vi "QTrkCheckForDLL.vi"   [LabVIEW 2011]
uses:
  QTrkDLL.vi
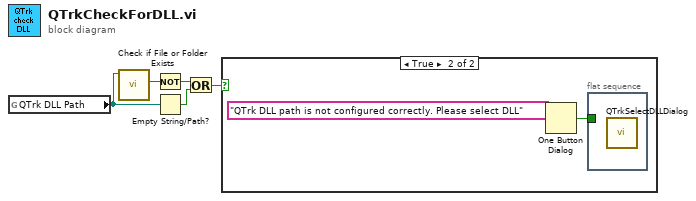
[diagram p0: block diagram]
diagram:
  n1 = global read "QTrkDLL.vi" "QTrk DLL Path"() -> (w5:path)
  n2 = call <vilib>:"Check if File or Folder Exists.vi"("path"=w5) -> ("file or folder exists?"=w3:bool)  [unwired: 8 in, 2 out]
  n3 = Not(x=w3) -> (.not. x?=w2:bool)
  n4 = Empty String/Path?(string/path=w5) -> (empty?=w1:bool)
  n5 = Or(x=w2, y=w1) -> (x .or. y?=w4:bool)
  n6 = case shown="True" w4 {
    frame False {
    }
    frame True {
      n7 = One Button Dialog(message="QTrk DLL path is not configured correctly. Please select DLL") -> (true=w6:bool)  [unwired: 1 in]
      n8 = flat-sequence {
        tunnel: w6 -> [_]
        frame #0 {
          n9 = call "QTrkSelectDLLDialog.vi"() -> ()  [unwired: 11 in, 1 out]
        }
      }
    }
  }
